vi "Format Errors.vi"(7 "Max Errors":bool, 10 "MultiErrors":T1[](array[typedef]), 11 "MultiError Formatter in":refnum<class "MultiError Formatter.lvclass">) -> (0 "error out":errorcluster)   [LabVIEW 2020, in "VolatusErrorUtilities.lvlib" / "MultiError Formatter.lvclass"]
uses:
  MultiError Formatter.lvclass
  MultiError.ctl
  VolatusErrorUtilities.lvlib
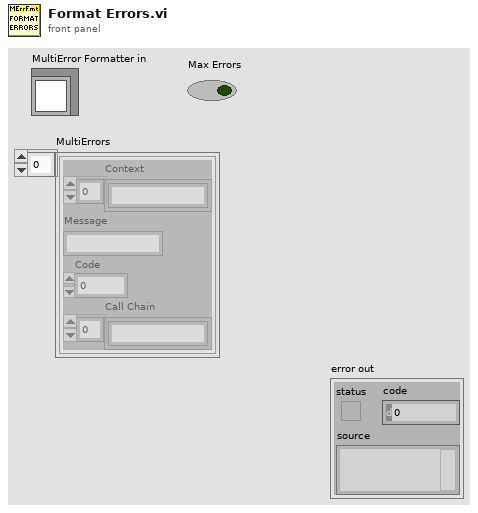
[diagram p1: front panel]
types:
  T1 = typedef "VolatusErrorUtilities.lvlib/MultiError.ctl" = cluster{"Context":string[], "Message":string, "Code":i32, "Call Chain":string[]}
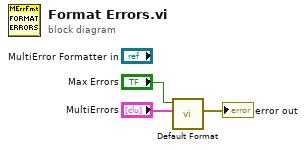
[diagram p0: block diagram]
diagram:
  n1 = call "Default Format.vi"("MultiErrors"="MultiErrors", "Max Errors"="Max Errors") -> ("error"=→"error out":errorcluster)  [unwired: 9 in]
